vi "Read.vi"(8 "error in (no error)":errorcluster, 10 "Channel Name":string, 11 "Data in":refnum<class "Data Server.lvclass">) -> (0 "error out":errorcluster, 1 "Found":bool, 2 "Data":string, 3 "Data out":refnum<class "Data Server.lvclass">)   [LabVIEW 2021, in "Veristandgrpc_server.lvlib" / "Data Server.lvclass"]
uses:
  Data Server.lvclass
  Data Server.lvclass/Data Server.ctl
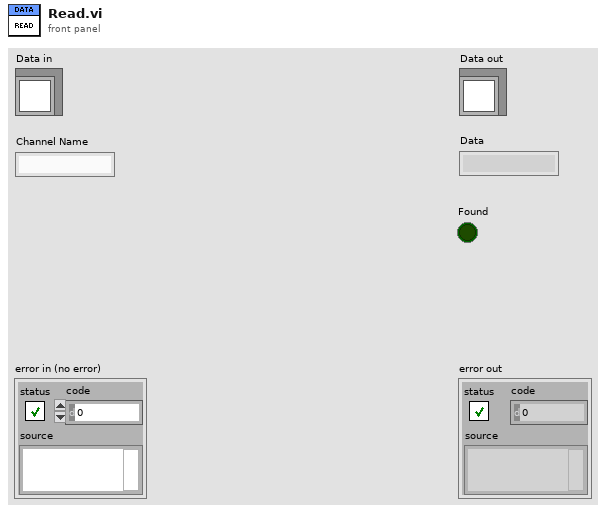
[diagram p1: front panel]
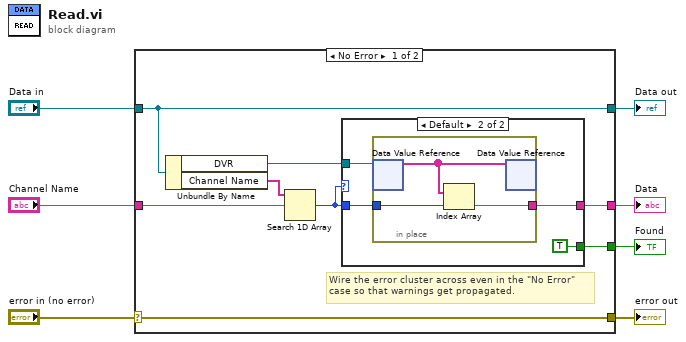
[diagram p0: block diagram]
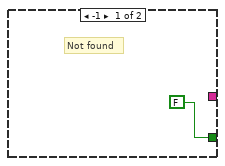
[diagram p2: hidden frame]
diagram:
  n1 = case shown="No Error" "error in (no error)" {
    selector: "error in (no error)" -> [w15 w25]
    tunnel: [w15 w25] -> w6
    tunnel: [w14 w24] -> w4
    tunnel: "Data in" -> [w14 w24]
    tunnel: "Channel Name" -> [w11 _]
    tunnel: [w9 _] -> w2
    tunnel: [w8 _] -> w1
    frame No Error {
      # "Wire the error cluster across even in the \"No Error\"\ncase so that warnings get propagated."
      n2 = Unbundle By Name(w14) -> ("DVR"=w13:refnum<data-value>, "Channel Name"=w12:string[])
      n3 = Search 1D Array(1D array=w12, element=w11) -> (index of element=w10:i32)  [unwired: 1 in]
      n4 = case shown="Default" w10 {
        tunnel: w13 -> [_ w20]
        tunnel: w10 -> [_ w19]
        tunnel: [FALSE TRUE] -> w9
        tunnel: [_ w17] -> w8
        frame -1 {
          # "Not found"
        }
        frame Default {
          n5 = in-place {
            in-place-border: w19 -> [w22]
            in-place-border: [w21] -> w17
            n6 = in-place-dvr #1(w20) -> (w23:string[])  [unwired: 1 out]
            n7 = Index Array(array=w23, index=w22) -> (element=w21:string)
            n8 = in-place-dvr #1(w23) -> ()  [unwired: 2 out]
          }
        }
      }
    }
    frame Error {
    }
  }
  "error out" <- w6
  "Data out" <- w4
  "Data" <- w1
  "Found" <- w2
